vi "core_h5_write_array_1d.vi"(7 "dataset name":string, 8 "error in (no error)":errorcluster, 9 "dim (index)":string="index", 10 "units (au)":string="au", 11 "h5 obj ref":i32) -> (0 "error out":errorcluster, 3 "h5 obj ref":i32)   [LabVIEW 2015]
uses:
  <vilib>/addons/h5labview2/base/lib_path.vi
  <vilib>/addons/h5labview2/base/H5Equery.vi
  <vilib>/addons/h5labview2/attrib/H5Awrite.llb/H5Awrite.xnode
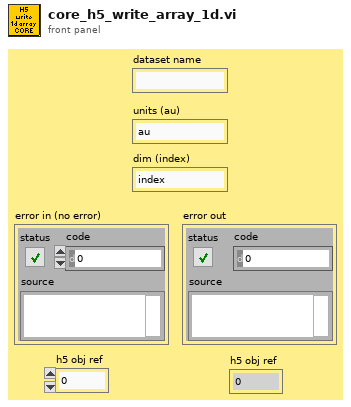
[diagram p1: front panel]
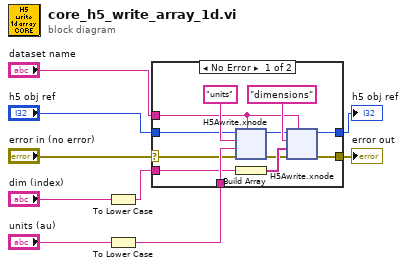
[diagram p0: block diagram]
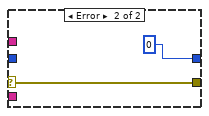
[diagram p2: hidden frame]
diagram:
  n1 = To Lower Case(string="dim (index)") -> (all lower case string=w2:string)
  n2 = To Lower Case(string="units (au)") -> (all lower case string=w4:string)
  n3 = case shown="No Error" "error in (no error)" {
    selector: "error in (no error)" -> [w10 w61]
    tunnel: "h5 obj ref" -> [w11 _]
    tunnel: w4 -> [w20 _]
    tunnel: w2 -> [w18 _]
    tunnel: "dataset name" -> [w14 _]
    tunnel: [w13 w61] -> w8
    tunnel: [w12 0] -> w7
    frame No Error {
      n4 = xnode "H5Awrite.xnode"("object name"=w14, "error in (no error)"=w10, "data"=w20, "attrib name"="units", "ref in"=w11) -> ("error out"=w16:errorcluster, "ref out"=w15:i32)  [unwired: 2 in, 1 out]
      n5 = Build Array(w18) -> (w17:string[])
      n6 = xnode "H5Awrite.xnode"("object name"=w14, "error in (no error)"=w16, "data"=w17, "attrib name"="dimensions", "ref in"=w15) -> ("error out"=w13:errorcluster, "ref out"=w12:i32)  [unwired: 2 in, 1 out]
    }
    frame Error {
    }
  }
  "error out" <- w8
  "h5 obj ref" <- w7
